vi "Variable Motor Power.vi"(1 "Power Off":bool, 2 "Power On":bool) -> (0 "Motor(s) Out":dbl)   [LabVIEW 2014]
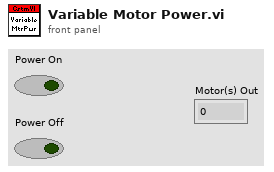
[diagram p1: front panel]
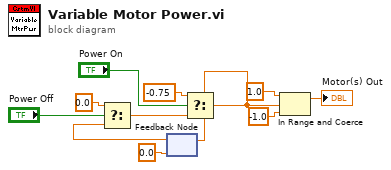
[diagram p0: block diagram]
diagram:
  n1 = feedback #1(0.0 ("t")) -> (w9:dbl)
  n2 = Select(t=0.0, s="Power Off", f=w9) -> (s? t:f=w8:dbl)
  n3 = Select(t=-0.75, s="Power On", f=w8) -> (s? t:f=w6:dbl)
  n4 = feedback-in #1(w6) -> ()
  n5 = In Range and Coerce(upper limit=1.0, x=w6, lower limit=-1.0) -> (coerced(x)=→"Motor(s) Out":dbl)  [unwired: 1 out]
